vi "Read Config Unitest.vi"(8 "error in (no error)":errorcluster, 11 "main ref":T1) -> (0 "error out":errorcluster)   [LabVIEW 2025]
uses:
  controls/LAB-IQ UI Data.ctl
  Traction Loop/Traction Receipe Enum.ctl
  Config file  FGV Unitest enum.ctl
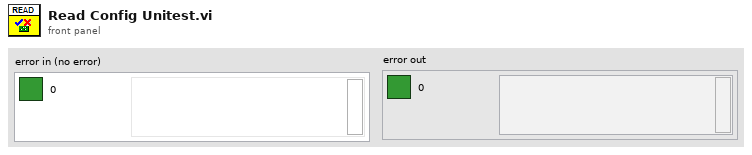
[diagram p1: front panel]
types:
  T1 = typedef "LAB-IQ UI Data.ctl" = cluster{"Main Home Screen":cluster{"GUI":refnum<vi>, "Platform Settings":refnum<vi>, "Configure":refnum<vi>, "Home":refnum<vi>, "EXIT":refnum<vi>, "service 2":refnum<vi>, "MainPage":refnum<vi>, "Analysis":refnum<vi>}, "Platform Settings":cluster{"mm/s  Surge":refnum<vi>, "Drive Error":refnum<vi>, "Disable Axis Jog Soft Limits":refnum<vi>, "mm/s  Sway":refnum<vi>, "Sway and Surge COM Status":refnum<vi>, "Heave COM Status":refnum<vi>, "Enable Platform":refnum<vi>, "Surge Forward Main":refnum<vi>, "Sway Right Main":refnum<vi>, "Sway Left Main":refnum<vi>, "Heave Down Main":refnum<vi>, "Heave Up main":refnum<vi>, "mm/s Heave":refnum<vi>, "mm/sec":refnum<vi>, "mm":refnum<vi>, "Surge Backward Main":refnum<vi>}, "Analysis Screen":cluster{"Analysis Home":refnum<vi>, "Surface Analysis":refnum<vi>, "Imaging":refnum<vi>, "Image Analysis":refnum<vi>, "Post Analysis":refnum<vi>}, "Config Screen":cluster{"Select Load Head":refnum<vi>, "Notes :":refnum<vi>, "FILE":refnum<vi>, "Sample ID :":refnum<vi>, "Operator ID :":refnum<vi>, "Operator Name :":refnum<vi>, "Auto":refnum<vi>}, "Motion Module":cluster{"zNL":refnum<vi>, "NL disp":refnum<vi>, "Rotary Tab":refnum<vi>, "Motion Direction:  3":refnum<vi>, "E.Velocity 2":refnum<vi>, "e.v/ssr 2":refnum<vi>, "Enter Fixed E.Velocity 2":refnum<vi>, "Enter Final SRR 2":refnum<vi>, "Enter initial SRR 2":refnum<vi>, "Enter Fixed SRR 2":refnum<vi>, "Enter the Final E.Velocity (m/s) 2":refnum<vi>, "Enter initial E.Velocity (m/s) 2":refnum<vi>, "Final Speed (RPM) 3":refnum<vi>, "Initial Speed (RPM) 2":refnum<vi>, "Enter the Final Velocity (m/s) 3":refnum<vi>, "Enter initial Velocity (m/s)  3":refnum<vi>, "Ramp Up 2":refnum<vi>, "TEST SELECTION":refnum<vi>, "SPEED SELECTION : ":refnum<vi>, "Angular Oscillation Set":refnum<vi>, "Traction":refnum<vi>, "Step Speed":refnum<vi>, "StepTable For Load-Speed":refnum<vi>, "StepTable For Speed":refnum<vi>, "Surge Forward MM":refnum<vi>, "Surge Backward MM":refnum<vi>, "M3 Image":refnum<vi>, "String 39":refnum<vi>, "Sway Left MM":refnum<vi>, "Sway Right MM":refnum<vi>, "Disable Axis Jog Soft Limits":refnum<vi>, "mm":refnum<vi>, "Heave Down MM":refnum<vi>, "Heave Up MM":refnum<vi>, "Wear Track Diameter (mm)":refnum<vi>, "Set WTD":refnum<vi>, "HomeScratch":refnum<vi>, "HomeRot":refnum<vi>, "PlaceModule":refnum<vi>, "Enter the Angle (Deg)":refnum<vi>, "Enter the Frequency (Hz)":refnum<vi>, "Motion Mode:":refnum<vi>, "LR Sway":refnum<vi>, "Rot Hor":refnum<vi>, "Scratch":refnum<vi>, "LR Cam":refnum<vi>, "MMBack":refnum<vi>, "MMNext":refnum<vi>, "Rot Ver":refnum<vi>, "Rotary Module Selection":refnum<vi>, "calculate rotary":refnum<vi>, "SPEED SELECTION : rotary":refnum<vi>, "Import 2":refnum<vi>, "Save 2":refnum<vi>, "File Path :  2":refnum<vi>, "String 45":refnum<vi>, "StepTable For Speed 3":refnum<vi>, "Enter the Speed(mm/sec)":refnum<vi>, "Enter the Speed(RPM)":refnum<vi>, "Enter Scratch Speed (mm/s):":refnum<vi>, "SwaySpeed Set":refnum<vi>, "Scartch Offset":refnum<vi>, "Motion type:":refnum<vi>, "HomeScratch 2":refnum<vi>, "Enter Scratch length (mm):":refnum<vi>, "Wear Track Diameter":refnum<vi>, "Rotary Speed Exced":refnum<vi>, "Scratch Mode":refnum<vi>, "No of Scratch":refnum<vi>}, "Environmental control":cluster{"Humidity  Status  3":refnum<vi>, "Low Temp  Status  2":refnum<vi>, "TK4 status 2":refnum<vi>, "Stage Temperature":refnum<vi>, "Sample Temperature":refnum<vi>, "Humidity (Amb)":refnum<vi>, "Clear List":refnum<vi>, "Add to list":refnum<vi>, "Wear":refnum<vi>, "Vibration":refnum<vi>, "Humidity (Chamber)":refnum<vi>, "Temperature (Chamber)":refnum<vi>, "ECR ":refnum<vi>, "Temperature (Amb)":refnum<vi>, "Microphone":refnum<vi>, "Acoustic Emission 3":refnum<vi>, "SNext":refnum<vi>, "APBack":refnum<vi>, "Enter the Temperature (°C):":refnum<vi>, "Enter the Stage \nTemperature (°C):":refnum<vi>, "Enter the Humidity (%Rh):":refnum<vi>, "Low Temp":refnum<vi>, "High Temp":refnum<vi>, "Humidity":refnum<vi>, "Sensors Picked":refnum<vi>}, "About Screen":cluster{"Password":refnum<vi>, "Home Service":refnum<vi>, "Advanced Setting":refnum<vi>, "About Tab":refnum<vi>, "ECR Port:":refnum<vi>, "Ramp Port:":refnum<vi>, "Installation/Replacement completed":refnum<vi>, "Loahead":refnum<vi>, "Heave and Surge COM Port:":refnum<vi>, "Sway COM Port:":refnum<vi>, "Temp Modbus:":refnum<vi>, "Humidity Port:":refnum<vi>, "Edit Gain Constants":refnum<vi>, "Save Gain Constants":refnum<vi>}, "Main Screen":cluster{"Main Screen Tab":refnum<vi>, "Angle and Frequency":refnum<vi>, "Stroke (mm)":refnum<vi>, "Angle (Deg)":refnum<vi>, "Main Speed Tab":refnum<vi>, "MTM MOTOR DISPLAY":refnum<vi>, "Disc Speed (m/sec)":refnum<vi>, "Ball Speed (m/sec)":refnum<vi>, "Disc Speed (RPM)":refnum<vi>, "Ball Speed (RPM)":refnum<vi>, "SPEED TAB":refnum<vi>, "Speed (m/sec)":refnum<vi>, "Set Speed (m/sec)":refnum<vi>, "Speed (RPM)":refnum<vi>, "Set Speed":refnum<vi>, "Time Tab":refnum<vi>, "Time ( HH:MM:SS ) 2":refnum<vi>, "Test Duration":refnum<vi>, "Test Duration 4":refnum<vi>, "TEST CYCLE":refnum<vi>, "TOTAL CYCLES":refnum<vi>, "Set Load (N)":refnum<vi>, "Temp Tabs":refnum<vi>, "Heater":refnum<vi>, "TK4 status":refnum<vi>, "ChamberTemp":refnum<vi>, "SetTmp":refnum<vi>, "Controller  Status":refnum<vi>, "ChamberTemp 2":refnum<vi>, "SetTmp 2":refnum<vi>, "Controller  Status 2":refnum<vi>, "ChamberTemp 3":refnum<vi>, "SetTmp 3":refnum<vi>, "Cooling":refnum<vi>, "Load Communication":refnum<vi>, "Ambient \nTemperature":refnum<vi>, "HumCOMStatus":refnum<vi>, "Ambient\n Humidity":refnum<vi>, "Freq (Hz)":refnum<vi>, "Load En":refnum<vi>, "NLt":refnum<vi>, "zNL 2":refnum<vi>, "Humidity On":refnum<vi>, "humidity disp":refnum<vi>, "Set Humidity":refnum<vi>, "NL disp 2":refnum<vi>, "Humidity On 2":refnum<vi>, "humidity disp 2":refnum<vi>, "Set Humidity 2":refnum<vi>, "NL disp 3":refnum<vi>, "AppLoadSeq scratch":refnum<vi>, "Stop Scratch":refnum<vi>, "ClrLog":refnum<vi>, "Trip Log":refnum<vi>, "STOP":refnum<vi>, "Start Test":refnum<vi>, "Test status":refnum<vi>, "AR Led":refnum<vi>, "Data":refnum<vi>, "Health":refnum<vi>, "Sway COM Status":refnum<vi>, "Heave COM Status":refnum<vi>, "Grp Tab":refnum<vi>, "Sub Graph":refnum<vi>, "SD (mm)":refnum<vi>, "Siliding distance Reset Graph":refnum<vi>, "SDGp":refnum<vi>, "Humidity Reset Graph":refnum<vi>, "HumrGp":refnum<vi>, "Acoustic Emission (mV)":refnum<vi>, "Aqucostic Reset Graph":refnum<vi>, "gACQUOS":refnum<vi>, "ECR RESET":refnum<vi>, "ECR":refnum<vi>, "Temperature Reset":refnum<vi>, "Acoustic Emission (mV) 2":refnum<vi>, "Aqucostic Reset Graph 2":refnum<vi>, "gACQUOS 2":refnum<vi>, "ECR RESET 2":refnum<vi>, "ECR 2":refnum<vi>, "Temperature Reset 2":refnum<vi>, "Temperature (deg c)":refnum<vi>, "Speed Reset Graph":refnum<vi>, "Speed Tab":refnum<vi>, "MTM DISC  SPEED":refnum<vi>, "MTM BALL SPEED":refnum<vi>, "speed mm/sec":refnum<vi>, "Hymidity":refnum<vi>, "Humidity Disable trip":refnum<vi>, "CoF Trip  2":refnum<vi>, "Depth Trip":refnum<vi>, "Weart Deapth":refnum<vi>, "Depth Reset Graph":refnum<vi>, "Weart":refnum<vi>, "Depthz":refnum<vi>, "Depth (µm)":refnum<vi>, "WearGp":refnum<vi>, "NL Trip 2":refnum<vi>, "Load pid":refnum<vi>, "Load Disable Trip":refnum<vi>, "Load Reset Graph":refnum<vi>, "NL Display 4":refnum<vi>, "Main Chart 3":refnum<vi>, "BACK":refnum<vi>, "Depth Trip 2":refnum<vi>, "COF TRIP ":refnum<vi>, "Friction Force (N)":refnum<vi>, "FF Reset Graph":refnum<vi>, "FF Disable Trip":refnum<vi>, "FF TRIP":refnum<vi>, "COF Disable Trip":refnum<vi>, "COF Reset Graph":refnum<vi>, "Start Test Temp":refnum<vi>, "zFF":refnum<vi>, "Friction Force (N) Graph":refnum<vi>, "Coefficient of Friction":refnum<vi>, "Scratch Start Test":refnum<vi>, "FF Tab":refnum<vi>, "Cyclic Friction Force (N)":refnum<vi>, "CZ FF":refnum<vi>, "Cyclic Friction Force (N) Graph":refnum<vi>, "Cyclic Coefficient of Friction":refnum<vi>, "Cyclic FF TRIP":refnum<vi>, "Cyclic FF Disable Trip":refnum<vi>, "cyclic COF Disable Trip":refnum<vi>, "cyclic COF TRIP":refnum<vi>, "cyclic COF Reset Graph":refnum<vi>, "Cyclic FF Reset Graph":refnum<vi>, "Test Trip":refnum<vi>, "Multi Scratch Pass":refnum<vi>, "Scratch Start Recording":refnum<vi>}, "Loading":cluster{"Indentation":refnum<vi>, "Reference Sample":refnum<vi>, "Load Cell Communication Slide":refnum<vi>, "com 3":refnum<vi>, "com":refnum<vi>, "DecaForce COM Status":refnum<vi>, "Update":refnum<vi>, "Clear 3":refnum<vi>, "seq":refnum<vi>, "Stribeck table":refnum<vi>, "Stribeck Table  For loading":refnum<vi>, "Loading Mode":refnum<vi>, "Enter the Final Load (N)":refnum<vi>, "Enter the CoF Trip":refnum<vi>, "Enter the Friction Force Trip":refnum<vi>, "Enter the Normal load Trip":refnum<vi>, "Enter the Load  (N)":refnum<vi>, "KiloForce":refnum<vi>, "DecaForce ":refnum<vi>, "MicroForce":refnum<vi>, "LHBack":refnum<vi>, "LHNext":refnum<vi>, "Enter the Loading Rate (N/min)":refnum<vi>, "Message":refnum<vi>, "Warning 2":refnum<vi>, "SSP 0.75":refnum<vi>, "SSP 0.5":refnum<vi>, "SSP 0.3":refnum<vi>, "Warning":refnum<vi>, "gui GIF":refnum<vi>, "Communication is established":refnum<vi>, "AppLoad 4":refnum<vi>, "Multipoint":refnum<vi>, "Load Selection":refnum<vi>}, "PID":cluster{"Ramp":refnum<vi>, "Vertical load (N)":refnum<vi>, "apply load":refnum<vi>, "apply load 2":refnum<vi>, "Enter ByPass Load":refnum<vi>, "Bypass Load":refnum<vi>, "gFF Rot":refnum<vi>}, "Config Parameters":cluster{"Tab Control 3":refnum<vi>, "Tab Control 19":refnum<vi>, "SAMPLES":refnum<vi>, "Re-initilaize":refnum<vi>, "Filter ON/OFF":refnum<vi>, "TracHomeSurgeOffsetCounts 10MM":refnum<vi>, "TracHomeSwayOffsetCounts 10MM":refnum<vi>, "Acoustic Emission:":refnum<vi>, "Apply Filter (FF)":refnum<vi>, "Filter% 2":refnum<vi>, "Apply Filter (Load)":refnum<vi>, "Filter% ":refnum<vi>, "Sway distance (mm)":refnum<vi>, "Surge distance (mm)":refnum<vi>, "DataSavingLoopDelay(ms)":refnum<vi>, "SAVE 2":refnum<vi>, "Enter Distance":refnum<vi>, "Sway Counts:":refnum<vi>, "Distance (mm): 3":refnum<vi>, "Surge Counts:":refnum<vi>, "Distance (mm): 2":refnum<vi>, "Distance (mm):":refnum<vi>, "Heave Counts:":refnum<vi>, "LRMHomeSurgeOffsetCounts":refnum<vi>, "LRMHomeSwayOffsetCounts":refnum<vi>, "TracHomeSurgeOffsetCounts 20MM":refnum<vi>, "TracHomeSwayOffsetCounts 20MM":refnum<vi>, "RotHomeSwayOffsetCounts":refnum<vi>, "RotHomeSurgeOffsetCounts":refnum<vi>, "Heave distance":refnum<vi>, "Zmm":refnum<vi>, "Heave Pulses/mm":refnum<vi>, "Surge Pulses/mm":refnum<vi>, "Sway Pulses/mm":refnum<vi>, "Heave Pitch":refnum<vi>, "Surge Pitch":refnum<vi>, "Sway Pitch":refnum<vi>, "Heave PPR":refnum<vi>, "Surge PPR":refnum<vi>, "Sway PPR":refnum<vi>, "Tab Control 5":refnum<vi>, "Tab Control 14":refnum<vi>, "Tab Control 26":refnum<vi>, "AE":refnum<vi>, "Heave Loop Delay":refnum<vi>, "Heave PID Speed":refnum<vi>, "Surge Jog Speed":refnum<vi>, "Heave Jog Speed":refnum<vi>, "Sway Loop Delay":refnum<vi>, "Sway PID Speed":refnum<vi>, "Sway Jog Speed":refnum<vi>, "DEPTH TRIP VALUE":refnum<vi>, "LOAD TRIP VALUE":refnum<vi>, "DEPTH TRIP   ENABLE":refnum<vi>, "LOAD TRIP  ENABLE":refnum<vi>, "CYCLIC FF TRIP VALUE":refnum<vi>, "FF TRIP VALUE":refnum<vi>, "CYCLIC CoF TRIP VALUE":refnum<vi>, "COF TRIP VALUE":refnum<vi>, "CYCLIC COF TRIP  ENABLE":refnum<vi>, "CYCLIC FF TRIP  ENABLE":refnum<vi>, "FF TRIP  ENABLE":refnum<vi>, "COF TRIP  ENABLE":refnum<vi>, "JOG TRIP LOAD VALUE (N)":refnum<vi>, "Rotary Vertical":refnum<vi>, "Traction":refnum<vi>, "Scratch":refnum<vi>, "LRM CAM":refnum<vi>, "Sway LRM":refnum<vi>, "Rotary Horizontal":refnum<vi>}, "Loading Com Port":cluster{"ClearAll":refnum<vi>, "Mz(Nm)":refnum<vi>, "My(Nm)":refnum<vi>, "Mx(Nm)":refnum<vi>, "Save Dwell":refnum<vi>, "Acq Delay (ms)":refnum<vi>, "Burst Delay (ms)":refnum<vi>, "model":refnum<vi>, "SN":refnum<vi>, "FFx(N)":refnum<vi>, "Sensor IP":refnum<vi>, "Port":refnum<vi>, "FFy(N)":refnum<vi>, "Load(N)":refnum<vi>, "delete Handle":refnum<vi>, "Create Handle":refnum<vi>, "ft_data":refnum<vi>, "ft_range":refnum<vi>, "ft_data 2":refnum<vi>, "stop 6":refnum<vi>, "running_flag":refnum<vi>, "ft_udp_handle":refnum<vi>, "get-data-return":refnum<vi>, "get-range-return":refnum<vi>, "zero-return":refnum<vi>, "filter-return":refnum<vi>, "initial-return":refnum<vi>, "deleteHandle-result":refnum<vi>, "Load Cell Temp":refnum<vi>, "Load Cell":refnum<vi>, "ZeroAll":refnum<vi>, "FORCE (N)":refnum<vi>, "TORQUE (N-m)":refnum<vi>, "Load Cell Link":refnum<vi>}, "Heave AND Surge":cluster{"SURGE POSE":refnum<vi>, "error out Read":refnum<vi>, "HEAVE POSE":refnum<vi>, "State":refnum<vi>, "Homed":refnum<vi>, "Sequence ID":refnum<vi>, "error out Write":refnum<vi>, "faultCode":refnum<vi>, "Ack ID":refnum<vi>, "SPEED":refnum<vi>, "Distance":refnum<vi>, "Mode Command":refnum<vi>, "Heave and Surge Read":refnum<vi>, "Read Heave Temp":refnum<vi>, "Spare 15":refnum<vi>, "Spare 14":refnum<vi>, "Spare 13":refnum<vi>, "Spare 12":refnum<vi>, "Spare 11":refnum<vi>, "Spare 10":refnum<vi>, "Spare 9":refnum<vi>, "Spare 8":refnum<vi>, "Spare 7":refnum<vi>, "Spare 4":refnum<vi>, "Spare 3":refnum<vi>, "Spare 2":refnum<vi>, "Humidity":refnum<vi>, "Temp":refnum<vi>, "Node Id":refnum<vi>, "Spare 1":refnum<vi>, "SPARE 4":refnum<vi>, "SPARE 3":refnum<vi>, "SPARE 2":refnum<vi>, "SPARE 1":refnum<vi>, "fwMajor":refnum<vi>, "fwMinor":refnum<vi>, "Manual Write":refnum<vi>, "Heave and Surge Write":refnum<vi>, "SPARE 5":refnum<vi>, "Reserved ":refnum<vi>, "SPARE 8":refnum<vi>, "SPARE 6":refnum<vi>, "SPARE 7":refnum<vi>, "SPARE 17":refnum<vi>, "SPARE 16":refnum<vi>, "SPARE 15":refnum<vi>, "SPARE 14":refnum<vi>, "SPARE 13":refnum<vi>, "SPARE 12":refnum<vi>, "SPARE 11":refnum<vi>, "SPARE 10":refnum<vi>, "SPARE 9":refnum<vi>, "System UPTIME":refnum<vi>, "Missed Packets":refnum<vi>, "faultCode Surge Right":refnum<vi>, "faultCode Surge Left":refnum<vi>, "faultCode Heave":refnum<vi>, "UPLINK HEAVE":refnum<vi>, "DOWNLINK HEAVE":refnum<vi>}, "New PID LOGIC":cluster{"Fine Tune Zone":refnum<vi>, "PID SDelay":refnum<vi>, "Max_pos_limit":refnum<vi>, "Min_pos_limit":refnum<vi>, "i_limit":refnum<vi>, "pct_scale":refnum<vi>, "Deadband":refnum<vi>, "Kd":refnum<vi>, "Ki":refnum<vi>, "Kp":refnum<vi>, "Current Position":refnum<vi>, "Set Load":refnum<vi>, "Current Load":refnum<vi>, "Pulse delta":refnum<vi>, "Init Step":refnum<vi>, "Max Step Linit":refnum<vi>, "min_deadband_floor":refnum<vi>, "dynamic_spindle_noise_scalar":refnum<vi>, "min_finetune_floor":refnum<vi>, "filter_alpha":refnum<vi>, "PID":refnum<vi>}, "SWAY ":cluster{"fwMajor":refnum<vi>, "Homed":refnum<vi>, "Rotary POSE":refnum<vi>, "State":refnum<vi>, "SWAY POSE":refnum<vi>, "Ack ID":refnum<vi>, "faultCode":refnum<vi>, "Node Id":refnum<vi>, "fwMinor":refnum<vi>, "Spare 6":refnum<vi>, "Spare 5":refnum<vi>, "Spare 4":refnum<vi>, "Spare 3":refnum<vi>, "Spare 2":refnum<vi>, "Spare 1":refnum<vi>, "Spare 7":refnum<vi>, "SPARE  5":refnum<vi>, "error out Write  SWAY ":refnum<vi>, "error out Read SWAY ":refnum<vi>, "Manual Write SWAY ":refnum<vi>, "SWAY WRITE":refnum<vi>, "SPARE  4":refnum<vi>, "SPARE  3":refnum<vi>, "SPARE 2":refnum<vi>, "SPARE 1":refnum<vi>, "Spare 15":refnum<vi>, "Spare 14":refnum<vi>, "Spare 13":refnum<vi>, "Spare 12":refnum<vi>, "Spare 11":refnum<vi>, "Spare 9":refnum<vi>, "Spare 8":refnum<vi>, "SPEED":refnum<vi>, "Distance":refnum<vi>, "Mode Command":refnum<vi>, "Sequence ID":refnum<vi>, "SWAY READ":refnum<vi>, "Spare 10":refnum<vi>, "Read SWAY Temp":refnum<vi>, "faultCode Sway ":refnum<vi>, "Missed Packets":refnum<vi>, "System UPTIME sway":refnum<vi>, "SPARE 6":refnum<vi>, "SPARE 7":refnum<vi>, "SPARE 9":refnum<vi>, "SPARE 11":refnum<vi>, "SPARE 10":refnum<vi>, "SPARE 8":refnum<vi>, "SPARE 13":refnum<vi>, "SPARE 12":refnum<vi>, "SPARE 17":refnum<vi>, "SPARE 16":refnum<vi>, "SPARE 15":refnum<vi>, "SPARE 14":refnum<vi>, "Reserved":refnum<vi>, "faultCode Rotary":refnum<vi>, "UPLINK SWAY":refnum<vi>, "DOWNLINK SWAY":refnum<vi>}, "Analysis Screen":cluster{"Analysis Home":refnum<vi>, "Refresh 2":refnum<vi>, "MEAN 4":refnum<vi>, "SD 4":refnum<vi>, "VARIANCE 4":refnum<vi>, "MEAN  3":refnum<vi>, "SD  3":refnum<vi>, "VARIANCE  3":refnum<vi>, "MEAN 2":refnum<vi>, "SD  2":refnum<vi>, "VARIANCE 2":refnum<vi>, "MEAN":refnum<vi>, "SD":refnum<vi>, "VARIANCE":refnum<vi>, "File 4 Discription":refnum<vi>, "OPEN 4":refnum<vi>, "File Name 4":refnum<vi>, "OPEN 3":refnum<vi>, "File 3 Discription":refnum<vi>, "File Name 3":refnum<vi>, "Y-AXIS":refnum<vi>, "X-AXIS":refnum<vi>, "XY Graph":refnum<vi>, "File Name 2":refnum<vi>, "File Name 1":refnum<vi>, "OPEN 2":refnum<vi>, "OPEN 1":refnum<vi>, "File 1 Discription ":refnum<vi>, "File 2 Discription":refnum<vi>, "Export":refnum<vi>, "File Format":refnum<vi>}, "Traction":cluster{"faultCode Traction 2":refnum<vi>, "faultCode Traction 1":refnum<vi>, "Missed Packets":refnum<vi>, "System UPTIME Traction":refnum<vi>, "SPARE 17":refnum<vi>, "SPARE 16":refnum<vi>, "SPARE 15":refnum<vi>, "SPARE 14":refnum<vi>, "SPARE 13":refnum<vi>, "SPARE 12":refnum<vi>, "SPARE 11":refnum<vi>, "SPARE 10":refnum<vi>, "SPARE 9":refnum<vi>, "SPARE 8":refnum<vi>, "SPARE 7":refnum<vi>, "SPARE 6":refnum<vi>, "Reserved":refnum<vi>, "SPARE  5":refnum<vi>, "Manual Write TRACTION":refnum<vi>, "TRACTION WRITE":refnum<vi>, "SPARE  4":refnum<vi>, "SPARE  3":refnum<vi>, "SPARE 2":refnum<vi>, "SPARE 1":refnum<vi>, "Spare 7":refnum<vi>, "Spare 6":refnum<vi>, "Spare 5":refnum<vi>, "Spare 4":refnum<vi>, "Spare 2":refnum<vi>, "Spare 1":refnum<vi>, "Node Id":refnum<vi>, "Read TRACTION Temp":refnum<vi>, "fwMinor":refnum<vi>, "fwMajor":refnum<vi>, "faultCode":refnum<vi>, "TRACTION POSE":refnum<vi>, "TRACTION POSE 2":refnum<vi>, "Homed":refnum<vi>, "State":refnum<vi>, "Ack ID":refnum<vi>, "SPEED":refnum<vi>, "Distance":refnum<vi>, "Mode Command":refnum<vi>, "Sequence ID":refnum<vi>, "error out Read TRACTION":refnum<vi>, "error out Write  TRACTION":refnum<vi>, "TRACTION READ":refnum<vi>, "Spare 3":refnum<vi>, "Downlink traction":refnum<vi>, "Uplink Traction":refnum<vi>}, "Traction reciepe":cluster{"SRR Sweep Range (%) Stribeck":refnum<vi>, "Traction Receipe":refnum<vi>, "Total Execution Time":refnum<vi>, "Total Steps":refnum<vi>, "Duration / Step (s)  Stribeck":refnum<vi>, "STRIBECK Fixed SRR List (%)":refnum<vi>, "Duration / Step (s) Traction":refnum<vi>, "SRR Sweep Range (%) traction":refnum<vi>, "Rolling Speed (mm/s)":refnum<vi>, "Temperature Stages (°C)":refnum<vi>, "Ball Load (N)":refnum<vi>, "Lubricant Name":refnum<vi>, "Profile File Name":refnum<vi>, "SET entrainment Velocity":refnum<vi>, "Test Array Size":refnum<vi>, "SRR INDEX [ STRIBECK]":refnum<vi>, "Stribeck Size":refnum<vi>, "SET SRR":refnum<vi>, "ELAPSED TIMER ":refnum<vi>, "BALL SET RPM":refnum<vi>, "DISC SET RPM":refnum<vi>, "SET LOAD":refnum<vi>, "TEMPERATURE READ":refnum<vi>, "SET TEMPERATURE":refnum<vi>, "Traction Size":refnum<vi>, "DISC SPEED (rpm)":refnum<vi>, "BALL SPEED (rpm)":refnum<vi>, "BALL WEAR TRACK":refnum<vi>, "DISC WEARTRACK":refnum<vi>, "SRR INDEX [ TRACTION]":refnum<vi>, "Start Index Type":refnum<vi>, "Enum - Menu":refnum<vi>, "Ball (mm/sec)":refnum<vi>, "Disc (mm/sec)":refnum<vi>}, "Traction Control":cluster{"HomeTraction":refnum<vi>, "Demo Mode Display":refnum<vi>, "Traction Message":refnum<vi>, "Traction Step Update Details":refnum<vi>, "Main Tab sequence for selection":refnum<vi>, "Ramp Tab":refnum<vi>, "e.v/ssr":refnum<vi>, "Enter Fixed E.Velocity":refnum<vi>, "Enter Final SRR":refnum<vi>, "Enter initial SRR":refnum<vi>, "Enter Fixed SRR":refnum<vi>, "Enter the Final E.Velocity (m/s)":refnum<vi>, "Enter initial E.Velocity (m/s)":refnum<vi>, "Ball WTD":refnum<vi>, "E.Velocity":refnum<vi>, "Enter the Final Velocity (m/s)":refnum<vi>, "Enter initial Velocity (m/s)":refnum<vi>, "Ramp Up   Disc":refnum<vi>, "Initial DiscSpeed (RPM)":refnum<vi>, "Final Speed (RPM) Ball":refnum<vi>, "Final Speed (RPM)":refnum<vi>, "Initial Speed (RPM) Ball":refnum<vi>, "Enter the Final Velocity (m/s) Ball":refnum<vi>, "Enter initial Velocity (m/s) Ball":refnum<vi>, "Ramp Up":refnum<vi>, "ExceedBallSpeed step":refnum<vi>, "ExceedDiscSpeed":refnum<vi>, "BallSpeed Exceed Indication":refnum<vi>, "Apply":refnum<vi>, "SPEED SELECTION : MTM":refnum<vi>, "SPEED SELECTION : MTM 2":refnum<vi>, "TEST SELECTION (MTM)":refnum<vi>, "MTM Test Selection":refnum<vi>, "File Path Tab":refnum<vi>, "File Path String":refnum<vi>, "Save":refnum<vi>, "Save  2":refnum<vi>, "Import ":refnum<vi>, "File Path :":refnum<vi>, "Step Sequence Indication Tab":refnum<vi>, "Step Sequence Indication":refnum<vi>, "Calculate Step":refnum<vi>, "StepTable":refnum<vi>, "ExceedDiscSpeed  Cinstant Speed":refnum<vi>, "ExceedBallSpeed Constant":refnum<vi>, "TEST SELECTION (MTM) 2":refnum<vi>, "SPEED SELECTION : MTM 3":refnum<vi>, "MTM Test Selection 2":refnum<vi>, "Enter the Speed (m/sec): ":refnum<vi>, "Enter the Speed (m/sec):  2":refnum<vi>, "Enter the Speed (RPM):":refnum<vi>, "Lower Spped ":refnum<vi>, "Upper":refnum<vi>, "Enter the Speed (RPM):Ball":refnum<vi>, "Disc Motion Direction: ":refnum<vi>, "Ball Motion Direction :":refnum<vi>, "Motion Mode: ":refnum<vi>, "Wear Track Diameter (mm) ":refnum<vi>, "Disc Speed Indicator":refnum<vi>, "ExceedBallSpeed":refnum<vi>}, "Acquostic":cluster{"Last Config Rejected ":refnum<vi>, "rx command count":refnum<vi>, "Current Filter Id":refnum<vi>, "Isolated Gain":refnum<vi>, "DAQ Status":refnum<vi>, "error out":refnum<vi>, "error in (no error)":refnum<vi>, "Uplink Packet":refnum<vi>, "data out":refnum<vi>, "Downlink Packet":refnum<vi>, "Gains":refnum<vi>, "Manual Write Acquostic":refnum<vi>, "Acoustic Graphs":refnum<vi>}}
  T2 = typedef "Config file  FGV Unitest enum.ctl" = enum16{"OPEN", "READ", "WRITE", "CLOSE"}
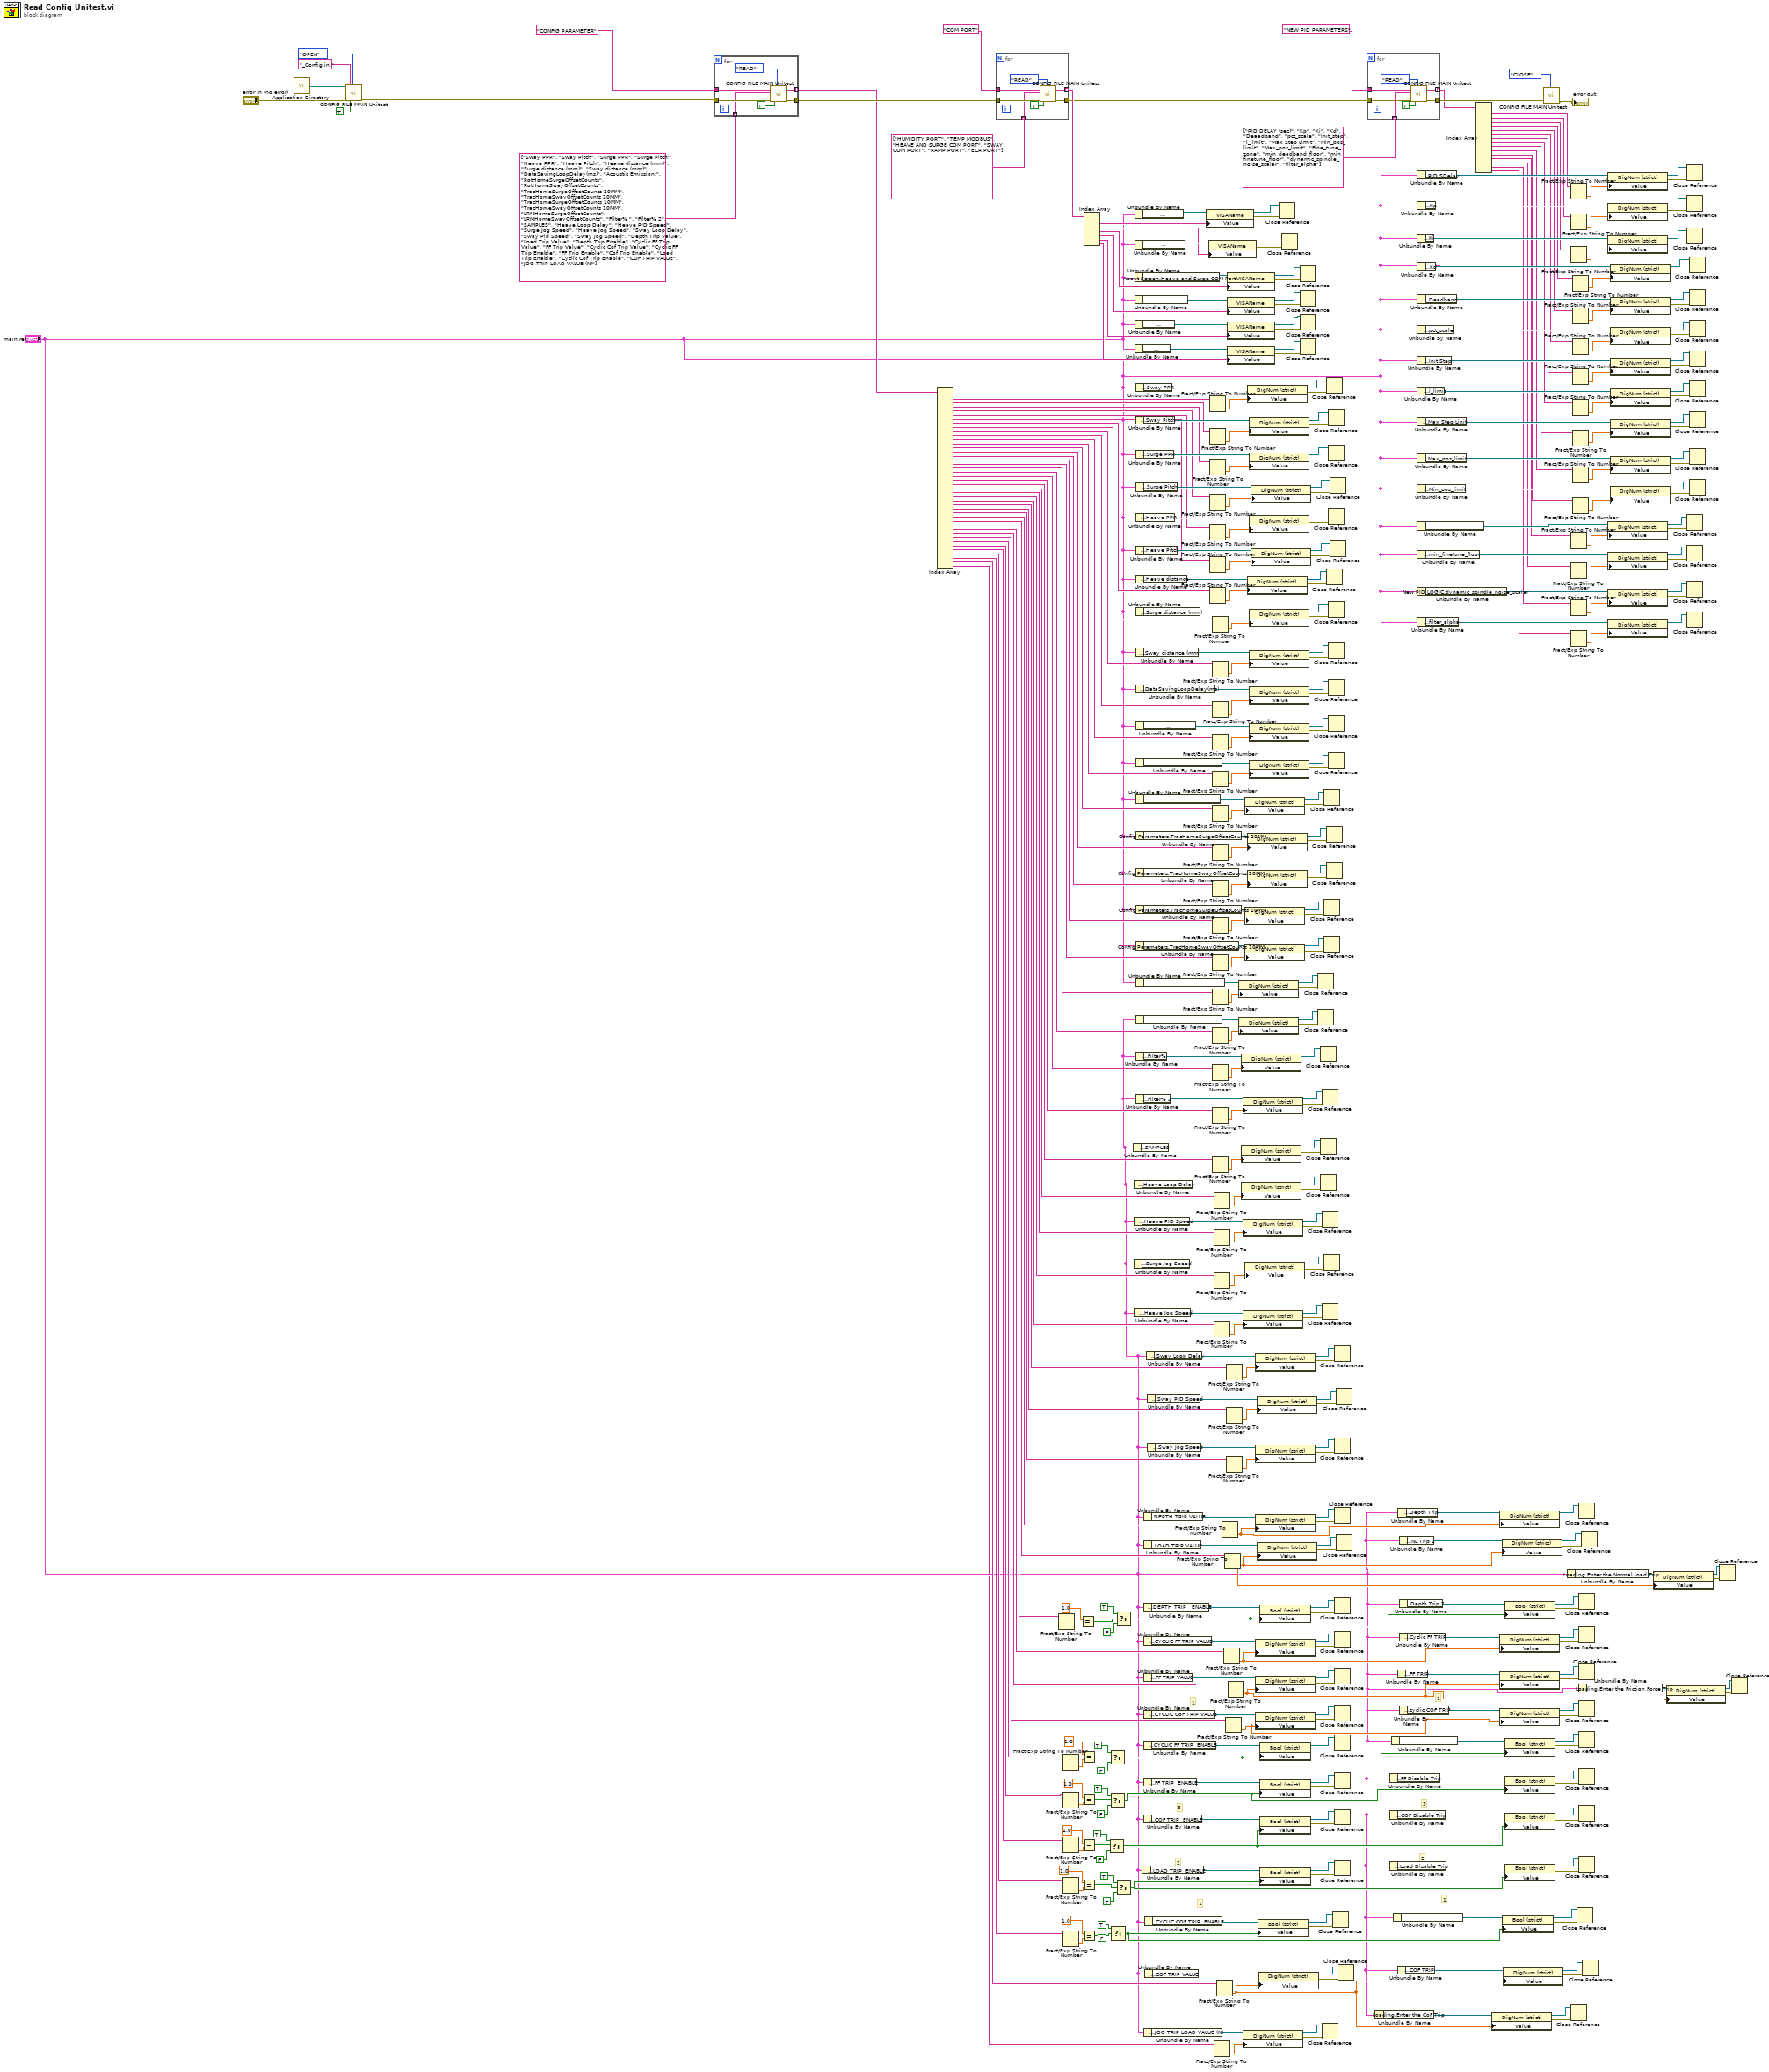
[diagram p0: block diagram]
diagram:
  # "3"
  # "2"
  # "1"
  # "1"
  # "3"
  # "2"
  # "1"
  # "1"
  n1 = call <vilib>:"Application Directory.vi"() -> ("Application Directory"=w401:path)
  n2 = call "CONFIG FILE MAIN Unitest.vi"("File Path"=w401, "error in"="error in (no error)", "file name"="_Config.ini", "PARAMETER/CONFIG"=TRUE, "Config Enum"=Config_file__FGV_Unitest_enum."OPEN") -> ("error out"=w400:errorcluster)  [unwired: 13 in, 1 out]
  n3 = for {
    tunnel: w400 -> [w412]
    tunnel: "CONFIG PARAMETER" ("WRITE /READ SECTION") -> [w411]
    tunnel: [w410] -> w398
    tunnel: string[] ["Sway PPR", "Sway Pitch", "Surge PPR", "Surge Pitch", "Heave PPR", "Heave Pitch", "Heave distance (mm)", "Surge distance (mm)", "Sway distance (mm)", "DataSavingLoopDelay(ms)", "Acoustic Emission:", "RotHomeSurgeOffsetCounts", "RotHomeSwayOffsetCounts", "TracHomeSurgeOffsetCounts 20MM", "TracHomeSwayOffsetCounts 20MM", "TracHomeSurgeOffsetCounts 10MM", "TracHomeSwayOffsetCounts 10MM", "LRMHomeSurgeOffsetCounts", "LRMHomeSwayOffsetCounts", "Filter% ", "Filter% 2", "SAMPLES", "Heave Loop Delay", "Heave PID Speed", "Surge Jog Speed", "Heave Jog Speed", "Sway Loop Delay", "Sway Pid Speed", "Sway Jog Speed", "Depth Trip Value", "Load Trip Value", "Depth Trip Enable", "Cyclic FF Trip Value", "FF Trip Value", "Cyclic Cof Trip Value", "Cyclic FF Trip Enable", "FF Trip Enable", "Cof Trip Enable", "Load Trip Enable", "Cyclic Cof Trip Enable", "COF TRIP VALUE", "JOG TRIP LOAD VALUE (N)"] -> [w407] mode=indexing
    tunnel: [w406] -> w302 mode=indexing
    n4 = call "CONFIG FILE MAIN Unitest.vi"("WRITE /READ SECTION"=w411, "READ KEY"=w407, "error in"=w412, "PARAMETER/CONFIG"=TRUE, "Config Enum"=Config_file__FGV_Unitest_enum."READ") -> ("READ VALUE"=w406:string, "error out"=w410:errorcluster)  [unwired: 13 in]
  }
  n5 = Index Array(array=w302) -> (element #1=w301:string, element #2=w300:string, element #3=w299:string, element #4=w298:string, element #5=w297:string, element #6=w296:string, element #7=w295:string, element #8=w294:string, element #9=w293:string, element #10=w292:string, element #11=w291:string, element #12=w290:string, element #13=w289:string, element #14=w288:string, element #15=w287:string, element #16=w286:string, element #17=w285:string, element #18=w284:string, element #19=w283:string, element #20=w282:string, element #21=w281:string, element #22=w280:string, element #23=w241:string, element #24=w240:string, element #25=w239:string, element #26=w238:string, element #27=w166:string, element #28=w165:string, element #29=w164:string, element #30=w114:string, element #31=w113:string, element #32=w112:string, element #33=w111:string, element #34=w110:string, element #35=w109:string, element #36=w108:string, element #37=w107:string, element #38=w106:string, element #39=w105:string, element #40=w104:string, element #41=w50:string, element #42=w2:string)  [unwired: 42 in]
  n6 = for {
    tunnel: w398 -> [w419]
    tunnel: "COM PORT" ("WRITE /READ SECTION") -> [w418]
    tunnel: [w417] -> w236
    tunnel: string[] ["HUMIDITY PORT", "TEMP MODBUS", "HEAVE AND SURGE COM PORT", "SWAY COM PORT", "RAMP PORT", "ECR PORT"] -> [w414] mode=indexing
    tunnel: [w413] -> w309 mode=indexing
    n7 = call "CONFIG FILE MAIN Unitest.vi"("WRITE /READ SECTION"=w418, "READ KEY"=w414, "error in"=w419, "PARAMETER/CONFIG"=TRUE, "Config Enum"=Config_file__FGV_Unitest_enum."READ") -> ("READ VALUE"=w413:string, "error out"=w417:errorcluster)  [unwired: 13 in]
  }
  n8 = Fract/Exp String To Number(string=w112) -> (number=w126:dbl)  [unwired: 3 in, 1 out]
  n9 = Fract/Exp String To Number(string=w108) -> (number=w127:dbl)  [unwired: 3 in, 1 out]
  n10 = Fract/Exp String To Number(string=w107) -> (number=w125:dbl)  [unwired: 3 in, 1 out]
  n11 = Fract/Exp String To Number(string=w106) -> (number=w124:dbl)  [unwired: 3 in, 1 out]
  n12 = Fract/Exp String To Number(string=w105) -> (number=w123:dbl)  [unwired: 3 in, 1 out]
  n13 = Fract/Exp String To Number(string=w104) -> (number=w122:dbl)  [unwired: 3 in, 1 out]
  n14 = Equal?(x=1.0, y=w126) -> (x = y?=w87:bool)
  n15 = Equal?(x=1.0, y=w127) -> (x = y?=w90:bool)
  n16 = Equal?(x=1.0, y=w125) -> (x = y?=w91:bool)
  n17 = Equal?(x=1.0, y=w124) -> (x = y?=w92:bool)
  n18 = Equal?(x=1.0, y=w123) -> (x = y?=w93:bool)
  n19 = Equal?(x=1.0, y=w122) -> (x = y?=w115:bool)
  n20 = Index Array(array=w309) -> (element #1=w308:string, element #2=w307:string, element #3=w306:string, element #4=w305:string, element #5=w304:string, element #6=w303:string)  [unwired: 6 in]
  n21 = Select(t=TRUE, s=w92, f=FALSE) -> (s? t:f=w47:bool)
  n22 = Select(t=TRUE, s=w90, f=FALSE) -> (s? t:f=w45:bool)
  n23 = Select(t=TRUE, s=w91, f=FALSE) -> (s? t:f=w46:bool)
  n24 = Select(t=TRUE, s=w115, f=FALSE) -> (s? t:f=w49:bool)
  n25 = Select(t=TRUE, s=w87, f=FALSE) -> (s? t:f=w42:bool)
  n26 = Select(t=TRUE, s=w93, f=FALSE) -> (s? t:f=w48:bool)
  n27 = Unbundle By Name("main ref") -> ("Config Parameters.SAMPLES"=w333:refnum<vi>)
  n28 = Unbundle By Name("main ref") -> ("Config Parameters.Heave Loop Delay"=w244:refnum<vi>)
  n29 = Unbundle By Name("main ref") -> ("Config Parameters.Heave PID Speed"=w245:refnum<vi>)
  n30 = Unbundle By Name("main ref") -> ("Config Parameters.Surge Jog Speed"=w249:refnum<vi>)
  n31 = Unbundle By Name("main ref") -> ("Config Parameters.Heave Jog Speed"=w250:refnum<vi>)
  n32 = Unbundle By Name("main ref") -> ("About Screen.Humidity Port:"=w327:refnum<vi>)
  n33 = Unbundle By Name("main ref") -> ("About Screen.Temp Modbus:"=w322:refnum<vi>)
  n34 = Unbundle By Name("main ref") -> ("About Screen.Heave and Surge COM Port:"=w321:refnum<vi>)
  n35 = Unbundle By Name("main ref") -> ("About Screen.Sway COM Port:"=w317:refnum<vi>)
  n36 = Unbundle By Name("main ref") -> ("About Screen.Ramp Port:"=w316:refnum<vi>)
  n37 = Unbundle By Name("main ref") -> ("About Screen.ECR Port:"=w313:refnum<vi>)
  n38 = Unbundle By Name("main ref") -> ("Config Parameters.Sway PPR"=w394:refnum<vi>)
  n39 = Unbundle By Name("main ref") -> ("Config Parameters.Sway Pitch"=w389:refnum<vi>)
  n40 = Unbundle By Name("main ref") -> ("Config Parameters.Surge PPR"=w383:refnum<vi>)
  n41 = Unbundle By Name("main ref") -> ("Config Parameters.Surge Pitch"=w388:refnum<vi>)
  n42 = Unbundle By Name("main ref") -> ("Config Parameters.Heave PPR"=w382:refnum<vi>)
  n43 = Unbundle By Name("main ref") -> ("Config Parameters.Heave Pitch"=w378:refnum<vi>)
  n44 = Unbundle By Name("main ref") -> ("Config Parameters.Heave distance"=w372:refnum<vi>)
  n45 = Unbundle By Name("main ref") -> ("Config Parameters.Surge distance (mm)"=w376:refnum<vi>)
  n46 = Unbundle By Name("main ref") -> ("Config Parameters.Sway distance (mm)"=w370:refnum<vi>)
  n47 = Unbundle By Name("main ref") -> ("Config Parameters.DataSavingLoopDelay(ms)"=w367:refnum<vi>)
  n48 = Unbundle By Name("main ref") -> ("Config Parameters.Acoustic Emission:"=w364:refnum<vi>)
  n49 = Unbundle By Name("main ref") -> ("Config Parameters.RotHomeSurgeOffsetCounts"=w361:refnum<vi>)
  n50 = Unbundle By Name("main ref") -> ("Config Parameters.RotHomeSwayOffsetCounts"=w358:refnum<vi>)
  n51 = Unbundle By Name("main ref") -> ("Config Parameters.TracHomeSurgeOffsetCounts 20MM"=w355:refnum<vi>)
  n52 = Unbundle By Name("main ref") -> ("Config Parameters.TracHomeSwayOffsetCounts 20MM"=w352:refnum<vi>)
  n53 = Unbundle By Name("main ref") -> ("Config Parameters.TracHomeSurgeOffsetCounts 10MM"=w348:refnum<vi>)
  n54 = Unbundle By Name("main ref") -> ("Config Parameters.TracHomeSwayOffsetCounts 10MM"=w351:refnum<vi>)
  n55 = Unbundle By Name("main ref") -> ("Config Parameters.LRMHomeSurgeOffsetCounts"=w342:refnum<vi>)
  n56 = Unbundle By Name("main ref") -> ("Config Parameters.LRMHomeSwayOffsetCounts"=w339:refnum<vi>)
  n57 = Unbundle By Name("main ref") -> ("Config Parameters.Filter%"=w338:refnum<vi>)
  n58 = Unbundle By Name("main ref") -> ("Config Parameters.Filter% 2"=w334:refnum<vi>)
  n59 = Unbundle By Name("main ref") -> ("Config Parameters.LOAD TRIP  ENABLE"=w136:refnum<vi>)
  n60 = Unbundle By Name("main ref") -> ("Config Parameters.DEPTH TRIP VALUE"=w137:refnum<vi>)
  n61 = Unbundle By Name("main ref") -> ("Config Parameters.LOAD TRIP VALUE"=w141:refnum<vi>)
  n62 = Unbundle By Name("main ref") -> ("Config Parameters.DEPTH TRIP   ENABLE"=w142:refnum<vi>)
  n63 = Unbundle By Name("main ref") -> ("Config Parameters.CYCLIC FF TRIP VALUE"=w148:refnum<vi>)
  n64 = Unbundle By Name("main ref") -> ("Config Parameters.FF TRIP VALUE"=w149:refnum<vi>)
  n65 = Unbundle By Name("main ref") -> ("Config Parameters.CYCLIC CoF TRIP VALUE"=w154:refnum<vi>)
  n66 = Unbundle By Name("main ref") -> ("Config Parameters.CYCLIC FF TRIP  ENABLE"=w155:refnum<vi>)
  n67 = Unbundle By Name("main ref") -> ("Config Parameters.FF TRIP  ENABLE"=w163:refnum<vi>)
  n68 = Unbundle By Name("main ref") -> ("Config Parameters.COF TRIP  ENABLE"=w158:refnum<vi>)
  n69 = Unbundle By Name("main ref") -> ("Config Parameters.JOG TRIP LOAD VALUE (N)"=w7:refnum<vi>)
  n70 = Unbundle By Name("main ref") -> ("Config Parameters.CYCLIC COF TRIP  ENABLE"=w131:refnum<vi>)
  n71 = Unbundle By Name("main ref") -> ("Config Parameters.COF TRIP VALUE"=w130:refnum<vi>)
  n72 = Unbundle By Name("main ref") -> ("Config Parameters.Sway Loop Delay"=w178:refnum<vi>)
  n73 = Unbundle By Name("main ref") -> ("Config Parameters.Sway PID Speed"=w174:refnum<vi>)
  n74 = Unbundle By Name("main ref") -> ("Config Parameters.Sway Jog Speed"=w173:refnum<vi>)
  n75 = property class="VISAName"(reference=w327, "Value"=w308) -> (reference out=w325:refnum<vi>, error out=w326:errorcluster)  [unwired: 1 in]
  n76 = property class="VISAName"(reference=w322, "Value"=w307) -> (reference out=w324:refnum<vi>, error out=w323:errorcluster)  [unwired: 1 in]
  n77 = Fract/Exp String To Number(string=w301) -> (number=w279:dbl)  [unwired: 3 in, 1 out]
  n78 = Fract/Exp String To Number(string=w300) -> (number=w278:dbl)  [unwired: 3 in, 1 out]
  n79 = Fract/Exp String To Number(string=w299) -> (number=w277:dbl)  [unwired: 3 in, 1 out]
  n80 = Fract/Exp String To Number(string=w298) -> (number=w276:dbl)  [unwired: 3 in, 1 out]
  n81 = Fract/Exp String To Number(string=w297) -> (number=w275:dbl)  [unwired: 3 in, 1 out]
  n82 = Fract/Exp String To Number(string=w296) -> (number=w274:dbl)  [unwired: 3 in, 1 out]
  n83 = Fract/Exp String To Number(string=w295) -> (number=w273:dbl)  [unwired: 3 in, 1 out]
  n84 = Fract/Exp String To Number(string=w294) -> (number=w272:dbl)  [unwired: 3 in, 1 out]
  n85 = Fract/Exp String To Number(string=w293) -> (number=w271:dbl)  [unwired: 3 in, 1 out]
  n86 = Fract/Exp String To Number(string=w292) -> (number=w270:dbl)  [unwired: 3 in, 1 out]
  n87 = Fract/Exp String To Number(string=w291) -> (number=w269:dbl)  [unwired: 3 in, 1 out]
  n88 = Fract/Exp String To Number(string=w290) -> (number=w268:dbl)  [unwired: 3 in, 1 out]
  n89 = Fract/Exp String To Number(string=w289) -> (number=w267:dbl)  [unwired: 3 in, 1 out]
  n90 = Fract/Exp String To Number(string=w288) -> (number=w266:dbl)  [unwired: 3 in, 1 out]
  n91 = Fract/Exp String To Number(string=w287) -> (number=w265:dbl)  [unwired: 3 in, 1 out]
  n92 = Fract/Exp String To Number(string=w286) -> (number=w264:dbl)  [unwired: 3 in, 1 out]
  n93 = Fract/Exp String To Number(string=w285) -> (number=w263:dbl)  [unwired: 3 in, 1 out]
  n94 = Fract/Exp String To Number(string=w284) -> (number=w262:dbl)  [unwired: 3 in, 1 out]
  n95 = Fract/Exp String To Number(string=w283) -> (number=w261:dbl)  [unwired: 3 in, 1 out]
  n96 = Fract/Exp String To Number(string=w282) -> (number=w260:dbl)  [unwired: 3 in, 1 out]
  n97 = Fract/Exp String To Number(string=w281) -> (number=w259:dbl)  [unwired: 3 in, 1 out]
  n98 = Fract/Exp String To Number(string=w280) -> (number=w258:dbl)  [unwired: 3 in, 1 out]
  n99 = Fract/Exp String To Number(string=w241) -> (number=w254:dbl)  [unwired: 3 in, 1 out]
  n100 = Fract/Exp String To Number(string=w240) -> (number=w255:dbl)  [unwired: 3 in, 1 out]
  n101 = Fract/Exp String To Number(string=w239) -> (number=w256:dbl)  [unwired: 3 in, 1 out]
  n102 = Fract/Exp String To Number(string=w238) -> (number=w257:dbl)  [unwired: 3 in, 1 out]
  n103 = Fract/Exp String To Number(string=w2) -> (number=w4:dbl)  [unwired: 3 in, 1 out]
  n104 = Fract/Exp String To Number(string=w50) -> (number=w37:dbl)  [unwired: 3 in, 1 out]
  n105 = Fract/Exp String To Number(string=w114) -> (number=w41:dbl)  [unwired: 3 in, 1 out]
  n106 = Fract/Exp String To Number(string=w111) -> (number=w43:dbl)  [unwired: 3 in, 1 out]
  n107 = Fract/Exp String To Number(string=w113) -> (number=w33:dbl)  [unwired: 3 in, 1 out]
  n108 = Fract/Exp String To Number(string=w109) -> (number=w44:dbl)  [unwired: 3 in, 1 out]
  n109 = Fract/Exp String To Number(string=w166) -> (number=w169:dbl)  [unwired: 3 in, 1 out]
  n110 = Fract/Exp String To Number(string=w165) -> (number=w168:dbl)  [unwired: 3 in, 1 out]
  n111 = Fract/Exp String To Number(string=w164) -> (number=w167:dbl)  [unwired: 3 in, 1 out]
  n112 = property class="VISAName"(reference=w321, "Value"=w306) -> (reference out=w319:refnum<vi>, error out=w320:errorcluster)  [unwired: 1 in]
  n113 = property class="VISAName"(reference=w317, "Value"=w305) -> (reference out=w312:refnum<vi>, error out=w318:errorcluster)  [unwired: 1 in]
  n114 = property class="VISAName"(reference=w316, "Value"=w304) -> (reference out=w311:refnum<vi>, error out=w315:errorcluster)  [unwired: 1 in]
  n115 = property class="VISAName"(reference=w313, "Value"=w303) -> (reference out=w310:refnum<vi>, error out=w314:errorcluster)  [unwired: 1 in]
  n116 = Fract/Exp String To Number(string=w110) -> (number=w29:dbl)  [unwired: 3 in, 1 out]
  n117 = property class="DigNum (strict)"(reference=w342, "Value"=w262) -> (reference out=w343:refnum<vi>, error out=w341:errorcluster)  [unwired: 1 in]
  n118 = property class="DigNum (strict)"(reference=w339, "Value"=w261) -> (reference out=w344:refnum<vi>, error out=w340:errorcluster)  [unwired: 1 in]
  n119 = property class="DigNum (strict)"(reference=w338, "Value"=w260) -> (reference out=w336:refnum<vi>, error out=w337:errorcluster)  [unwired: 1 in]
  n120 = property class="DigNum (strict)"(reference=w333, "Value"=w258) -> (reference out=w331:refnum<vi>, error out=w332:errorcluster)  [unwired: 1 in]
  n121 = property class="DigNum (strict)"(reference=w244, "Value"=w254) -> (reference out=w242:refnum<vi>, error out=w243:errorcluster)  [unwired: 1 in]
  n122 = property class="DigNum (strict)"(reference=w334, "Value"=w259) -> (reference out=w330:refnum<vi>, error out=w335:errorcluster)  [unwired: 1 in]
  n123 = property class="DigNum (strict)"(reference=w245, "Value"=w255) -> (reference out=w247:refnum<vi>, error out=w246:errorcluster)  [unwired: 1 in]
  n124 = property class="DigNum (strict)"(reference=w250, "Value"=w257) -> (reference out=w252:refnum<vi>, error out=w251:errorcluster)  [unwired: 1 in]
  n125 = property class="DigNum (strict)"(reference=w7, "Value"=w4) -> (reference out=w5:refnum<vi>, error out=w6:errorcluster)  [unwired: 1 in]
  n126 = property class="DigNum (strict)"(reference=w358, "Value"=w267) -> (reference out=w357:refnum<vi>, error out=w359:errorcluster)  [unwired: 1 in]
  n127 = property class="DigNum (strict)"(reference=w348, "Value"=w264) -> (reference out=w346:refnum<vi>, error out=w349:errorcluster)  [unwired: 1 in]
  n128 = property class="DigNum (strict)"(reference=w351, "Value"=w263) -> (reference out=w345:refnum<vi>, error out=w350:errorcluster)  [unwired: 1 in]
  n129 = property class="DigNum (strict)"(reference=w249, "Value"=w256) -> (reference out=w253:refnum<vi>, error out=w248:errorcluster)  [unwired: 1 in]
  n130 = property class="DigNum (strict)"(reference=w394, "Value"=w279) -> (reference out=w392:refnum<vi>, error out=w393:errorcluster)  [unwired: 1 in]
  n131 = property class="DigNum (strict)"(reference=w372, "Value"=w273) -> (reference out=w329:refnum<vi>, error out=w373:errorcluster)  [unwired: 1 in]
  n132 = property class="DigNum (strict)"(reference=w355, "Value"=w266) -> (reference out=w356:refnum<vi>, error out=w354:errorcluster)  [unwired: 1 in]
  n133 = property class="DigNum (strict)"(reference=w352, "Value"=w265) -> (reference out=w347:refnum<vi>, error out=w353:errorcluster)  [unwired: 1 in]
  n134 = property class="DigNum (strict)"(reference=w389, "Value"=w278) -> (reference out=w391:refnum<vi>, error out=w390:errorcluster)  [unwired: 1 in]
  n135 = property class="DigNum (strict)"(reference=w383, "Value"=w277) -> (reference out=w385:refnum<vi>, error out=w384:errorcluster)  [unwired: 1 in]
  n136 = property class="DigNum (strict)"(reference=w382, "Value"=w275) -> (reference out=w377:refnum<vi>, error out=w381:errorcluster)  [unwired: 1 in]
  n137 = property class="DigNum (strict)"(reference=w376, "Value"=w272) -> (reference out=w374:refnum<vi>, error out=w375:errorcluster)  [unwired: 1 in]
  n138 = property class="DigNum (strict)"(reference=w370, "Value"=w271) -> (reference out=w369:refnum<vi>, error out=w371:errorcluster)  [unwired: 1 in]
  n139 = property class="DigNum (strict)"(reference=w367, "Value"=w270) -> (reference out=w368:refnum<vi>, error out=w366:errorcluster)  [unwired: 1 in]
  n140 = property class="DigNum (strict)"(reference=w364, "Value"=w269) -> (reference out=w363:refnum<vi>, error out=w365:errorcluster)  [unwired: 1 in]
  n141 = property class="DigNum (strict)"(reference=w361, "Value"=w268) -> (reference out=w362:refnum<vi>, error out=w360:errorcluster)  [unwired: 1 in]
  n142 = property class="DigNum (strict)"(reference=w388, "Value"=w276) -> (reference out=w386:refnum<vi>, error out=w387:errorcluster)  [unwired: 1 in]
  n143 = property class="DigNum (strict)"(reference=w378, "Value"=w274) -> (reference out=w380:refnum<vi>, error out=w379:errorcluster)  [unwired: 1 in]
  n144 = property class="DigNum (strict)"(reference=w178, "Value"=w169) -> (reference out=w176:refnum<vi>, error out=w177:errorcluster)  [unwired: 1 in]
  n145 = property class="DigNum (strict)"(reference=w173, "Value"=w167) -> (reference out=w171:refnum<vi>, error out=w172:errorcluster)  [unwired: 1 in]
  n146 = property class="DigNum (strict)"(reference=w137, "Value"=w41) -> (reference out=w139:refnum<vi>, error out=w138:errorcluster)  [unwired: 1 in]
  n147 = property class="DigNum (strict)"(reference=w148, "Value"=w43) -> (reference out=w146:refnum<vi>, error out=w147:errorcluster)  [unwired: 1 in]
  n148 = property class="DigNum (strict)"(reference=w149, "Value"=w29) -> (reference out=w151:refnum<vi>, error out=w150:errorcluster)  [unwired: 1 in]
  n149 = property class="DigNum (strict)"(reference=w154, "Value"=w44) -> (reference out=w152:refnum<vi>, error out=w153:errorcluster)  [unwired: 1 in]
  n150 = property class="DigNum (strict)"(reference=w174, "Value"=w168) -> (reference out=w170:refnum<vi>, error out=w175:errorcluster)  [unwired: 1 in]
  n151 = property class="DigNum (strict)"(reference=w141, "Value"=w33) -> (reference out=w145:refnum<vi>, error out=w140:errorcluster)  [unwired: 1 in]
  n152 = property class="Bool (strict)"(reference=w131, "Value"=w49) -> (reference out=w133:refnum<vi>, error out=w132:errorcluster)  [unwired: 1 in]
  n153 = property class="DigNum (strict)"(reference=w130, "Value"=w37) -> (reference out=w128:refnum<vi>, error out=w129:errorcluster)  [unwired: 1 in]
  n154 = property class="Bool (strict)"(reference=w142, "Value"=w42) -> (reference out=w144:refnum<vi>, error out=w143:errorcluster)  [unwired: 1 in]
  n155 = property class="Bool (strict)"(reference=w155, "Value"=w45) -> (reference out=w157:refnum<vi>, error out=w156:errorcluster)  [unwired: 1 in]
  n156 = property class="Bool (strict)"(reference=w163, "Value"=w46) -> (reference out=w161:refnum<vi>, error out=w162:errorcluster)  [unwired: 1 in]
  n157 = property class="Bool (strict)"(reference=w158, "Value"=w47) -> (reference out=w160:refnum<vi>, error out=w159:errorcluster)  [unwired: 1 in]
  n158 = property class="Bool (strict)"(reference=w136, "Value"=w48) -> (reference out=w134:refnum<vi>, error out=w135:errorcluster)  [unwired: 1 in]
  n159 = Close Reference(reference=w325, error in (no error)=w326) -> ()  [unwired: 1 out]
  n160 = Close Reference(reference=w324, error in (no error)=w323) -> ()  [unwired: 1 out]
  n161 = Close Reference(reference=w319, error in (no error)=w320) -> ()  [unwired: 1 out]
  n162 = Close Reference(reference=w312, error in (no error)=w318) -> ()  [unwired: 1 out]
  n163 = Close Reference(reference=w311, error in (no error)=w315) -> ()  [unwired: 1 out]
  n164 = Close Reference(reference=w310, error in (no error)=w314) -> ()  [unwired: 1 out]
  n165 = Close Reference(reference=w343, error in (no error)=w341) -> ()  [unwired: 1 out]
  n166 = Close Reference(reference=w344, error in (no error)=w340) -> ()  [unwired: 1 out]
  n167 = Close Reference(reference=w336, error in (no error)=w337) -> ()  [unwired: 1 out]
  n168 = Close Reference(reference=w331, error in (no error)=w332) -> ()  [unwired: 1 out]
  n169 = Close Reference(reference=w242, error in (no error)=w243) -> ()  [unwired: 1 out]
  n170 = Close Reference(reference=w330, error in (no error)=w335) -> ()  [unwired: 1 out]
  n171 = Close Reference(reference=w247, error in (no error)=w246) -> ()  [unwired: 1 out]
  n172 = Close Reference(reference=w252, error in (no error)=w251) -> ()  [unwired: 1 out]
  n173 = Close Reference(reference=w5, error in (no error)=w6) -> ()  [unwired: 1 out]
  n174 = Close Reference(reference=w357, error in (no error)=w359) -> ()  [unwired: 1 out]
  n175 = Close Reference(reference=w346, error in (no error)=w349) -> ()  [unwired: 1 out]
  n176 = Close Reference(reference=w345, error in (no error)=w350) -> ()  [unwired: 1 out]
  n177 = Close Reference(reference=w253, error in (no error)=w248) -> ()  [unwired: 1 out]
  n178 = Close Reference(reference=w392, error in (no error)=w393) -> ()  [unwired: 1 out]
  n179 = Close Reference(reference=w329, error in (no error)=w373) -> ()  [unwired: 1 out]
  n180 = Close Reference(reference=w356, error in (no error)=w354) -> ()  [unwired: 1 out]
  n181 = Close Reference(reference=w347, error in (no error)=w353) -> ()  [unwired: 1 out]
  n182 = Close Reference(reference=w391, error in (no error)=w390) -> ()  [unwired: 1 out]
  n183 = Close Reference(reference=w385, error in (no error)=w384) -> ()  [unwired: 1 out]
  n184 = Close Reference(reference=w377, error in (no error)=w381) -> ()  [unwired: 1 out]
  n185 = Close Reference(reference=w374, error in (no error)=w375) -> ()  [unwired: 1 out]
  n186 = Close Reference(reference=w369, error in (no error)=w371) -> ()  [unwired: 1 out]
  n187 = Close Reference(reference=w368, error in (no error)=w366) -> ()  [unwired: 1 out]
  n188 = Close Reference(reference=w363, error in (no error)=w365) -> ()  [unwired: 1 out]
  n189 = Close Reference(reference=w362, error in (no error)=w360) -> ()  [unwired: 1 out]
  n190 = Close Reference(reference=w386, error in (no error)=w387) -> ()  [unwired: 1 out]
  n191 = Close Reference(reference=w380, error in (no error)=w379) -> ()  [unwired: 1 out]
  n192 = Close Reference(reference=w133, error in (no error)=w132) -> ()  [unwired: 1 out]
  n193 = Close Reference(reference=w176, error in (no error)=w177) -> ()  [unwired: 1 out]
  n194 = Close Reference(reference=w171, error in (no error)=w172) -> ()  [unwired: 1 out]
  n195 = Close Reference(reference=w139, error in (no error)=w138) -> ()  [unwired: 1 out]
  n196 = Close Reference(reference=w144, error in (no error)=w143) -> ()  [unwired: 1 out]
  n197 = Close Reference(reference=w146, error in (no error)=w147) -> ()  [unwired: 1 out]
  n198 = Close Reference(reference=w151, error in (no error)=w150) -> ()  [unwired: 1 out]
  n199 = Close Reference(reference=w152, error in (no error)=w153) -> ()  [unwired: 1 out]
  n200 = Close Reference(reference=w157, error in (no error)=w156) -> ()  [unwired: 1 out]
  n201 = Close Reference(reference=w161, error in (no error)=w162) -> ()  [unwired: 1 out]
  n202 = Close Reference(reference=w160, error in (no error)=w159) -> ()  [unwired: 1 out]
  n203 = Close Reference(reference=w134, error in (no error)=w135) -> ()  [unwired: 1 out]
  n204 = Close Reference(reference=w170, error in (no error)=w175) -> ()  [unwired: 1 out]
  n205 = Close Reference(reference=w145, error in (no error)=w140) -> ()  [unwired: 1 out]
  n206 = Close Reference(reference=w128, error in (no error)=w129) -> ()  [unwired: 1 out]
  n207 = for {
    tunnel: "NEW PID PARAMETERS" ("WRITE /READ SECTION") -> [w426]
    tunnel: [w425] -> w235
    tunnel: string[] ["PID DELAY (sec)", "Kp", "Ki", "Kd", "Deaadband", "pct_scale", "Init_step", "i_limit", "Max Step Limit", "Min_pos_limit", "Max_pos_limit", "Fine_tune_zone", "min_deadband_floor", "min_finetune_floor", "dynamic_spindle_noise_scalar", "filter_alpha"] -> [w422] mode=indexing
    tunnel: [w421] -> w208 mode=indexing
    tunnel: w236 -> [w420]
    n208 = call "CONFIG FILE MAIN Unitest.vi"("WRITE /READ SECTION"=w426, "READ KEY"=w422, "error in"=w420, "PARAMETER/CONFIG"=TRUE, "Config Enum"=Config_file__FGV_Unitest_enum."READ") -> ("READ VALUE"=w421:string, "error out"=w425:errorcluster)  [unwired: 13 in]
  }
  n209 = Unbundle By Name("main ref") -> ("Loading.Enter the CoF Trip"=w40:refnum<vi>)
  n210 = Unbundle By Name("main ref") -> ("Main Screen.Load Disable Trip"=w78:refnum<vi>)
  n211 = Unbundle By Name("main ref") -> ("Main Screen.FF Disable Trip"=w51:refnum<vi>)
  n212 = Unbundle By Name("main ref") -> ("Main Screen.COF Disable Trip"=w56:refnum<vi>)
  n213 = Unbundle By Name("main ref") -> ("Main Screen.Cyclic FF Disable Trip"=w59:refnum<vi>)
  n214 = Unbundle By Name("main ref") -> ("Main Screen.cyclic COF Disable Trip"=w83:refnum<vi>)
  n215 = Unbundle By Name("main ref") -> ("Main Screen.FF TRIP"=w65:refnum<vi>)
  n216 = Unbundle By Name("main ref") -> ("Main Screen.COF TRIP"=w84:refnum<vi>)
  n217 = Unbundle By Name("main ref") -> ("Main Screen.Depth Trip"=w77:refnum<vi>)
  n218 = Unbundle By Name("main ref") -> ("Main Screen.Depth Trip 2"=w72:refnum<vi>)
  n219 = Unbundle By Name("main ref") -> ("Main Screen.Cyclic FF TRIP"=w66:refnum<vi>)
  n220 = Unbundle By Name("main ref") -> ("Main Screen.cyclic COF TRIP"=w60:refnum<vi>)
  n221 = Unbundle By Name("main ref") -> ("Main Screen.NL Trip 2"=w73:refnum<vi>)
  n222 = Unbundle By Name("main ref") -> ("New PID LOGIC.PID SDelay"=w232:refnum<vi>)
  n223 = Unbundle By Name("main ref") -> ("New PID LOGIC.Kp"=w231:refnum<vi>)
  n224 = Unbundle By Name("main ref") -> ("New PID LOGIC.Ki"=w226:refnum<vi>)
  n225 = Unbundle By Name("main ref") -> ("New PID LOGIC.Kd"=w225:refnum<vi>)
  n226 = Unbundle By Name("main ref") -> ("New PID LOGIC.Deadband"=w221:refnum<vi>)
  n227 = Unbundle By Name("main ref") -> ("New PID LOGIC.pct_scale"=w220:refnum<vi>)
  n228 = Unbundle By Name("main ref") -> ("New PID LOGIC.Init Step"=w217:refnum<vi>)
  n229 = Unbundle By Name("main ref") -> ("New PID LOGIC.i_limit"=w216:refnum<vi>)
  n230 = Unbundle By Name("main ref") -> ("New PID LOGIC.Max Step Linit"=w213:refnum<vi>)
  n231 = Unbundle By Name("main ref") -> ("New PID LOGIC.Max_pos_limit"=w211:refnum<vi>)
  n232 = Unbundle By Name("main ref") -> ("New PID LOGIC.Min_pos_limit"=w210:refnum<vi>)
  n233 = Unbundle By Name("main ref") -> ("New PID LOGIC.min_deadband_floor"=w28:refnum<vi>)
  n234 = Unbundle By Name("main ref") -> ("New PID LOGIC.min_finetune_floor"=w25:refnum<vi>)
  n235 = Unbundle By Name("main ref") -> ("New PID LOGIC.dynamic_spindle_noise_scalar"=w23:refnum<vi>)
  n236 = Unbundle By Name("main ref") -> ("New PID LOGIC.filter_alpha"=w22:refnum<vi>)
  n237 = Index Array(array=w208) -> (element #1=w207:string, element #2=w206:string, element #3=w203:string, element #4=w202:string, element #5=w201:string, element #6=w200:string, element #7=w195:string, element #8=w194:string, element #9=w193:string, element #10=w192:string, element #11=w191:string, element #12=w13:string, element #13=w12:string, element #14=w11:string, element #15=w10:string)  [unwired: 15 in]
  n238 = property class="DigNum (strict)"(reference=w40, "Value"=w37) -> (reference out=w38:refnum<vi>, error out=w39:errorcluster)  [unwired: 1 in]
  n239 = property class="DigNum (strict)"(reference=w77, "Value"=w41) -> (reference out=w75:refnum<vi>, error out=w76:errorcluster)  [unwired: 1 in]
  n240 = property class="DigNum (strict)"(reference=w66, "Value"=w43) -> (reference out=w68:refnum<vi>, error out=w67:errorcluster)  [unwired: 1 in]
  n241 = property class="DigNum (strict)"(reference=w65, "Value"=w29) -> (reference out=w63:refnum<vi>, error out=w64:errorcluster)  [unwired: 1 in]
  n242 = property class="DigNum (strict)"(reference=w60, "Value"=w44) -> (reference out=w62:refnum<vi>, error out=w61:errorcluster)  [unwired: 1 in]
  n243 = property class="DigNum (strict)"(reference=w73, "Value"=w33) -> (reference out=w69:refnum<vi>, error out=w74:errorcluster)  [unwired: 1 in]
  n244 = property class="Bool (strict)"(reference=w83, "Value"=w49) -> (reference out=w81:refnum<vi>, error out=w82:errorcluster)  [unwired: 1 in]
  n245 = property class="DigNum (strict)"(reference=w84, "Value"=w37) -> (reference out=w86:refnum<vi>, error out=w85:errorcluster)  [unwired: 1 in]
  n246 = property class="Bool (strict)"(reference=w72, "Value"=w42) -> (reference out=w70:refnum<vi>, error out=w71:errorcluster)  [unwired: 1 in]
  n247 = property class="Bool (strict)"(reference=w59, "Value"=w45) -> (reference out=w57:refnum<vi>, error out=w58:errorcluster)  [unwired: 1 in]
  n248 = property class="Bool (strict)"(reference=w51, "Value"=w46) -> (reference out=w53:refnum<vi>, error out=w52:errorcluster)  [unwired: 1 in]
  n249 = property class="Bool (strict)"(reference=w56, "Value"=w47) -> (reference out=w54:refnum<vi>, error out=w55:errorcluster)  [unwired: 1 in]
  n250 = property class="Bool (strict)"(reference=w78, "Value"=w48) -> (reference out=w80:refnum<vi>, error out=w79:errorcluster)  [unwired: 1 in]
  n251 = call "CONFIG FILE MAIN Unitest.vi"("error in"=w235, "Config Enum"=Config_file__FGV_Unitest_enum."CLOSE") -> ("error out"=→"error out":errorcluster)  [unwired: 16 in, 1 out]
  n252 = Unbundle By Name("main ref") -> ("Loading.Enter the Normal load Trip"=w36:refnum<vi>)
  n253 = Fract/Exp String To Number(string=w207) -> (number=w205:dbl)  [unwired: 3 in, 1 out]
  n254 = Fract/Exp String To Number(string=w206) -> (number=w204:dbl)  [unwired: 3 in, 1 out]
  n255 = Fract/Exp String To Number(string=w203) -> (number=w199:dbl)  [unwired: 3 in, 1 out]
  n256 = Fract/Exp String To Number(string=w13) -> (number=w20:dbl)  [unwired: 3 in, 1 out]
  n257 = Fract/Exp String To Number(string=w12) -> (number=w19:dbl)  [unwired: 3 in, 1 out]
  n258 = Fract/Exp String To Number(string=w11) -> (number=w18:dbl)  [unwired: 3 in, 1 out]
  n259 = Fract/Exp String To Number(string=w10) -> (number=w17:dbl)  [unwired: 3 in, 1 out]
  n260 = Close Reference(reference=w38, error in (no error)=w39) -> ()  [unwired: 1 out]
  n261 = Fract/Exp String To Number(string=w202) -> (number=w198:dbl)  [unwired: 3 in, 1 out]
  n262 = Fract/Exp String To Number(string=w201) -> (number=w197:dbl)  [unwired: 3 in, 1 out]
  n263 = Fract/Exp String To Number(string=w200) -> (number=w196:dbl)  [unwired: 3 in, 1 out]
  n264 = Fract/Exp String To Number(string=w195) -> (number=w190:dbl)  [unwired: 3 in, 1 out]
  n265 = Fract/Exp String To Number(string=w194) -> (number=w189:dbl)  [unwired: 3 in, 1 out]
  n266 = Fract/Exp String To Number(string=w193) -> (number=w188:dbl)  [unwired: 3 in, 1 out]
  n267 = Fract/Exp String To Number(string=w192) -> (number=w187:dbl)  [unwired: 3 in, 1 out]
  n268 = Fract/Exp String To Number(string=w191) -> (number=w186:dbl)  [unwired: 3 in, 1 out]
  n269 = Close Reference(reference=w81, error in (no error)=w82) -> ()  [unwired: 1 out]
  n270 = Unbundle By Name("main ref") -> ("Loading.Enter the Friction Force Trip"=w32:refnum<vi>)
  n271 = Close Reference(reference=w75, error in (no error)=w76) -> ()  [unwired: 1 out]
  n272 = Close Reference(reference=w70, error in (no error)=w71) -> ()  [unwired: 1 out]
  n273 = Close Reference(reference=w68, error in (no error)=w67) -> ()  [unwired: 1 out]
  n274 = Close Reference(reference=w63, error in (no error)=w64) -> ()  [unwired: 1 out]
  n275 = Close Reference(reference=w62, error in (no error)=w61) -> ()  [unwired: 1 out]
  n276 = Close Reference(reference=w57, error in (no error)=w58) -> ()  [unwired: 1 out]
  n277 = Close Reference(reference=w53, error in (no error)=w52) -> ()  [unwired: 1 out]
  n278 = Close Reference(reference=w54, error in (no error)=w55) -> ()  [unwired: 1 out]
  n279 = Close Reference(reference=w80, error in (no error)=w79) -> ()  [unwired: 1 out]
  n280 = Close Reference(reference=w69, error in (no error)=w74) -> ()  [unwired: 1 out]
  n281 = Close Reference(reference=w86, error in (no error)=w85) -> ()  [unwired: 1 out]
  n282 = property class="DigNum (strict)"(reference=w232, "Value"=w205) -> (reference out=w234:refnum<vi>, error out=w233:errorcluster)  [unwired: 1 in]
  n283 = property class="DigNum (strict)"(reference=w231, "Value"=w204) -> (reference out=w229:refnum<vi>, error out=w230:errorcluster)  [unwired: 1 in]
  n284 = property class="DigNum (strict)"(reference=w226, "Value"=w199) -> (reference out=w228:refnum<vi>, error out=w227:errorcluster)  [unwired: 1 in]
  n285 = property class="DigNum (strict)"(reference=w28, "Value"=w20) -> (reference out=w9:refnum<vi>, error out=w27:errorcluster)  [unwired: 1 in]
  n286 = property class="DigNum (strict)"(reference=w25, "Value"=w19) -> (reference out=w16:refnum<vi>, error out=w26:errorcluster)  [unwired: 1 in]
  n287 = property class="DigNum (strict)"(reference=w23, "Value"=w18) -> (reference out=w15:refnum<vi>, error out=w24:errorcluster)  [unwired: 1 in]
  n288 = property class="DigNum (strict)"(reference=w22, "Value"=w17) -> (reference out=w14:refnum<vi>, error out=w21:errorcluster)  [unwired: 1 in]
  n289 = property class="DigNum (strict)"(reference=w225, "Value"=w198) -> (reference out=w223:refnum<vi>, error out=w224:errorcluster)  [unwired: 1 in]
  n290 = property class="DigNum (strict)"(reference=w221, "Value"=w197) -> (reference out=w184:refnum<vi>, error out=w222:errorcluster)  [unwired: 1 in]
  n291 = property class="DigNum (strict)"(reference=w220, "Value"=w196) -> (reference out=w185:refnum<vi>, error out=w219:errorcluster)  [unwired: 1 in]
  n292 = property class="DigNum (strict)"(reference=w217, "Value"=w190) -> (reference out=w183:refnum<vi>, error out=w218:errorcluster)  [unwired: 1 in]
  n293 = property class="DigNum (strict)"(reference=w216, "Value"=w189) -> (reference out=w182:refnum<vi>, error out=w215:errorcluster)  [unwired: 1 in]
  n294 = property class="DigNum (strict)"(reference=w213, "Value"=w188) -> (reference out=w181:refnum<vi>, error out=w214:errorcluster)  [unwired: 1 in]
  n295 = property class="DigNum (strict)"(reference=w211, "Value"=w187) -> (reference out=w180:refnum<vi>, error out=w212:errorcluster)  [unwired: 1 in]
  n296 = property class="DigNum (strict)"(reference=w210, "Value"=w186) -> (reference out=w179:refnum<vi>, error out=w209:errorcluster)  [unwired: 1 in]
  n297 = property class="DigNum (strict)"(reference=w36, "Value"=w33) -> (reference out=w34:refnum<vi>, error out=w35:errorcluster)  [unwired: 1 in]
  n298 = property class="DigNum (strict)"(reference=w32, "Value"=w29) -> (reference out=w30:refnum<vi>, error out=w31:errorcluster)  [unwired: 1 in]
  n299 = Close Reference(reference=w234, error in (no error)=w233) -> ()  [unwired: 1 out]
  n300 = Close Reference(reference=w229, error in (no error)=w230) -> ()  [unwired: 1 out]
  n301 = Close Reference(reference=w228, error in (no error)=w227) -> ()  [unwired: 1 out]
  n302 = Close Reference(reference=w9, error in (no error)=w27) -> ()  [unwired: 1 out]
  n303 = Close Reference(reference=w16, error in (no error)=w26) -> ()  [unwired: 1 out]
  n304 = Close Reference(reference=w15, error in (no error)=w24) -> ()  [unwired: 1 out]
  n305 = Close Reference(reference=w14, error in (no error)=w21) -> ()  [unwired: 1 out]
  n306 = Close Reference(reference=w223, error in (no error)=w224) -> ()  [unwired: 1 out]
  n307 = Close Reference(reference=w184, error in (no error)=w222) -> ()  [unwired: 1 out]
  n308 = Close Reference(reference=w185, error in (no error)=w219) -> ()  [unwired: 1 out]
  n309 = Close Reference(reference=w183, error in (no error)=w218) -> ()  [unwired: 1 out]
  n310 = Close Reference(reference=w182, error in (no error)=w215) -> ()  [unwired: 1 out]
  n311 = Close Reference(reference=w181, error in (no error)=w214) -> ()  [unwired: 1 out]
  n312 = Close Reference(reference=w180, error in (no error)=w212) -> ()  [unwired: 1 out]
  n313 = Close Reference(reference=w179, error in (no error)=w209) -> ()  [unwired: 1 out]
  n314 = Close Reference(reference=w34, error in (no error)=w35) -> ()  [unwired: 1 out]
  n315 = Close Reference(reference=w30, error in (no error)=w31) -> ()  [unwired: 1 out]
